vi "zmq_poll_array.vi"(4 "error in":errorcluster, 5 "timeout":i32, 6 "poll type":T1[](array[typedef]), 7 "sockets":refnum<class "zmq_socket.lvclass">[](array[class])) -> (0 "error out":errorcluster, 1 "timed out?":bool, 2 "nevents":i32, 3 "polled events":T1[](array[typedef]))   [LabVIEW 2020, in "zeromq.lvlib" / "zmq_socket.lvclass"]
doc: "Poll multiple sockets and for events. Blocks for <b>timeout</b> milliseconds or until an event occur on any of the given <b>sockets</b>. If no event happens, then <b>timed out?</b> is True.\n\nThe array <b>poll type</b> contains events to look for, and <b>must</b> contain a value for each socket provided. The enumeration contains the events to poll for.\n\nIf <b>timeout</b> is zero, the function returns immediately, regardless of whether any events are waiting. If <b>timeout</b> is negative, the function will block until an event occurs.\n\nDetailed API documentation: http://api.zeromq.org/3-2:zmq-poll"
uses:
  zmq_socket.lvclass
  poll_type.ctl
  zmq_socket.lvclass/zmq_socket.ctl
  Error Cluster From Error Code.vi
  zeromq.lvlib
panel:
  # "ØMQ"
  # "labview"
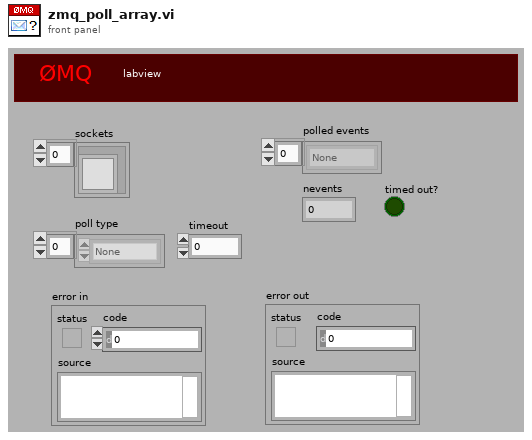
[diagram p1: front panel]
types:
  T1 = typedef "zeromq.lvlib/poll_type.ctl" = enum16{"None", "In", "Out", "In/Out"}
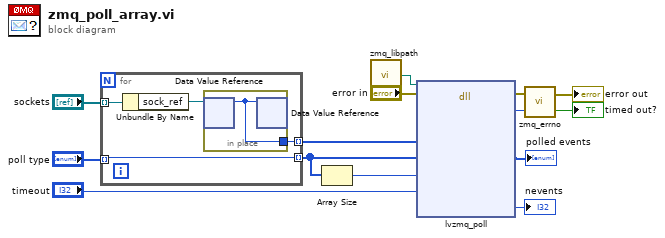
[diagram p0: block diagram]
diagram:
  n1 = for {
    tunnel: "sockets" -> [w18] mode=indexing
    tunnel: [w16] -> w6 mode=indexing
    tunnel: [w17] -> w3 mode=indexing
    tunnel: "poll type" -> [w17] mode=indexing
    n2 = Unbundle By Name(w18) -> ("sock_ref"=w15:refnum<data-value>)
    n3 = in-place {
      in-place-border: [w19] -> w16
      n4 = in-place-dvr #1(w15) -> (w19:u64)  [unwired: 1 out]
      n5 = in-place-dvr #1(w19) -> ()  [unwired: 2 out]
    }
  }
  n6 = Array Size(array=w3) -> (size(s)=w2:i32)
  n7 = call "zmq_libpath.vi"() -> ("path"=w1:path)
  n8 = dll-call lib="?" fn="lvzmq_poll" ("zmq_labview.dll:lvzmq_socket")(path in=w1, error in="error in", "socket"=w6, "evt"=w3, "n"=w2, "timeout"="timeout") -> (error out=w14:errorcluster, "return type"=w13:i32, "evt"=→"polled events":i32[], "nevents"=→"nevents":u32)  [unwired: 7 in, 1 out]
  n9 = call "zmq_errno.vi"("retval"=w13, "error in"=w14) -> ("again?"=→"timed out?":bool, "error out"=→"error out":errorcluster)
